vi "Apply Jerk Limit.vi"(8 "dt":dbl, 9 "jMax":dbl, 10 "aTarget":dbl, 11 "aCurrent":dbl) -> (3 "aNext":dbl)   [LabVIEW 2025]
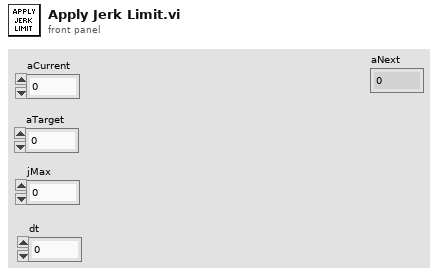
[diagram p1: front panel]
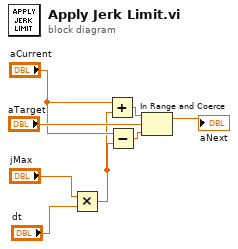
[diagram p0: block diagram]
diagram:
  n1 = Multiply(x="jMax", y="dt") -> (x*y=w3:dbl)
  n2 = Add(x="aCurrent", y=w3) -> (x+y=w2:dbl)
  n3 = Subtract(x="aCurrent", y=w3) -> (x-y=w5:dbl)
  n4 = In Range and Coerce(upper limit=w2, x="aTarget", lower limit=w5) -> (coerced(x)=→"aNext":dbl)  [unwired: 1 out]
